vi "RadWag Continuous Read.vi"() -> ()   [LabVIEW 2017]
doc: "This VI runs contnious read of mass walue from connected balance. Depending on settings result can be returned in balance current unit or in base unit (g). Also balance can return mass immediately or after displayed result became stable."
uses:
  <instrlib>/Prev/RadWag Continuous Read Folder/RadWag balances and scales.lvlib
panel:
  out "Mass":dbl format="%.2g"
  in  "Serial Configuration":T1={"Baud Rate"=9600, "Parity"=0, "Data Bits"=7, "Stop Bits"=10, "Flow Control"=0} {"Flow Control" items=["None", "XON/XOFF", "RTS/CTS", "XON/XOFF & RTS/CTS", "DTR/DSR", "XON/XOFF & DTR/DSR"]; "Stop Bits" items=["1.0"=10, "1.5"=15, "2.0"=20]; "Data Bits" items=["7"=7, "8"=8]; "Parity" items=["None", "Odd", "Even", "Mark", "Space"]; "Baud Rate" items=["300"=300, "600"=600, "1200"=1200, "2400"=2400, "4800"=4800, "9600"=9600, "19200"=19200]}
  in  "Actual Unit (F: Base unit)":bool
  in  "Immediately  (F: Wait for stable result)":bool
  out "Unit":string
  in  "VISA resource name":refnum<visa-resource-name>
  in  "Stop":bool
  out "Mass chart":dbl(graph)
  # "(c) 2014 Przemysłowy Instytut Automatyki i Pomiarów PIAP.  ALL RIGHTS RESERVED."
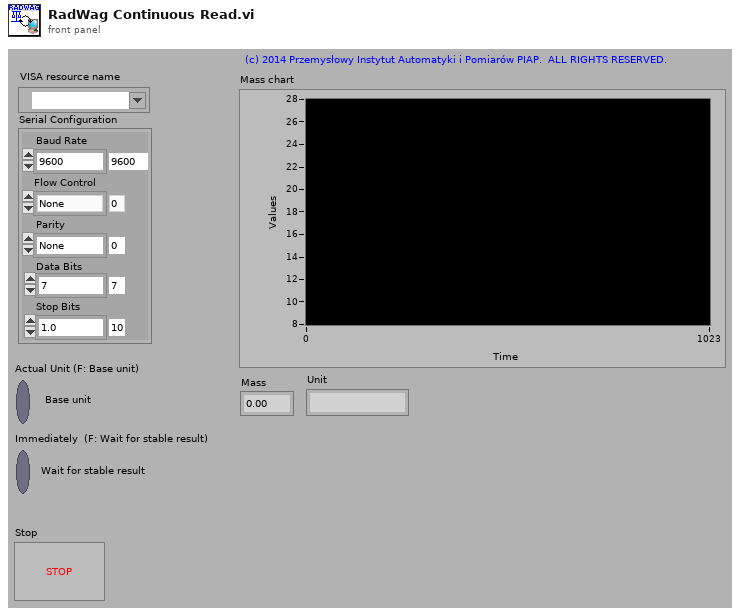
[diagram p1: front panel]
types:
  T1 = cluster{"Baud Rate":u32, "Parity":u16, "Data Bits":u16, "Stop Bits":u16, "Flow Control":u16}
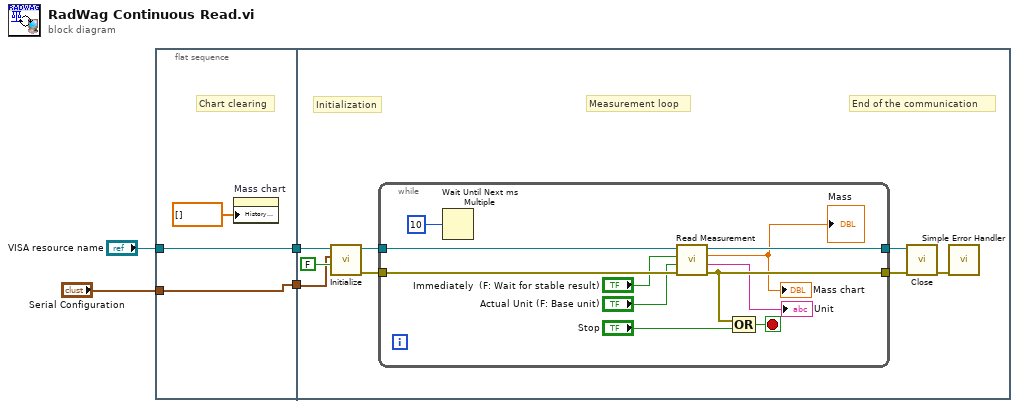
[diagram p0: block diagram]
diagram:
  n1 = flat-sequence {
    tunnel: [w6] -> w4
    tunnel: "VISA resource name" -> [w6]
    tunnel: [w5] -> w2
    tunnel: "Serial Configuration" -> [w5]
    tunnel: w4 -> [w10]
    tunnel: w2 -> [w8]
    frame #0 {
      # "Chart clearing"
      n2 = property on="Mass chart" class="WFChart (strict)"("History Data"=dbl[] []) -> ()  [unwired: 2 in, 2 out]
    }
    frame #1 {
      # "End of the communication"
      # "Measurement loop"
      # "Initialization"
      n3 = call <instrlib>:"Initialize.vi"("ID Query (True)"=FALSE, "Serial Configuration"=w8, "VISA resource name"=w10) -> ("error out"=w14:errorcluster, "VISA resource name out"=w15:refnum<visa-resource-name>)  [unwired: 7 in]
      n4 = while {
        tunnel: w15 -> [w25]
        tunnel: w14 -> [w26]
        tunnel: [w24] -> w12
        tunnel: [w23] -> w11
        stop <- w22 stop-if-true
        n5 = Wait Until Next ms Multiple(millisecond multiple=u32 10) -> ()  [unwired: 1 out]
        n6 = call <instrlib>:"Read Measurement.vi"("error in (no error)"=w26, "Actual Unit (F: Base unit)"="Actual Unit (F: Base unit)", "Immediately  (F: Wait for stable result)"="Immediately  (F: Wait for stable result)", "VISA resource name"=w25) -> ("error out"=w23:errorcluster, "Unit"=→"Unit":string, "Value"=→"Mass chart" →"Mass":dbl, "VISA resource name out"=w24:refnum<visa-resource-name>)  [unwired: 3 in, 1 out]
        n7 = Compound Arithmetic op=OR(w23, "Stop") -> (w22:bool)
      }
      n8 = call <instrlib>:"Close.vi"("error in (no error)"=w11, "VISA resource name"=w12) -> ("error out"=w13:errorcluster)  [unwired: 9 in]
      n9 = call <vilib>:"Simple Error Handler.vi"("error in (no error)"=w13) -> ()  [unwired: 4 in, 5 out]
    }
  }
